vi "Abort Sequence.vi"(8 "error in (no error)":errorcluster, 10 "Sequence Name":string, 11 "Sequencing Control in":refnum<class "Sequencing Control.lvclass">) -> (0 "error out":errorcluster, 3 "Sequencing Control out":refnum<class "Sequencing Control.lvclass">)   [LabVIEW 2020, in "VolatusSeqGUI.lvlib" / "Sequencing Control.lvclass"]
uses:
  Sequencing Control.lvclass
  Sequencing Control.lvclass/Sequencing Control.ctl
  <vilib>/httpClient/LabVIEWHTTPClient.lvlib
  <vilib>/httpClient/MultipartData.ctl
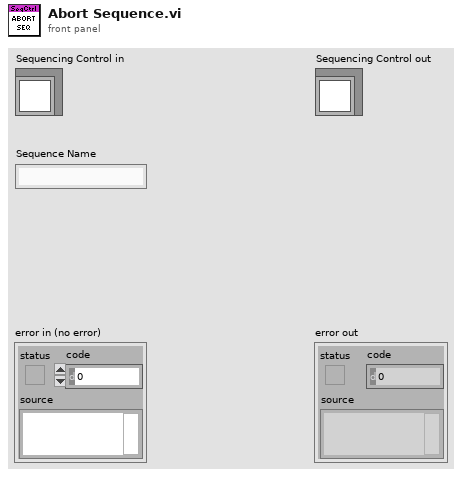
[diagram p1: front panel]
types:
  T1 = typedef "LabVIEWHTTPClient.lvlib/MultipartData.ctl" = cluster{"Name":string, "Value":string, "File":path, "Filename":string, "MIME type":string}
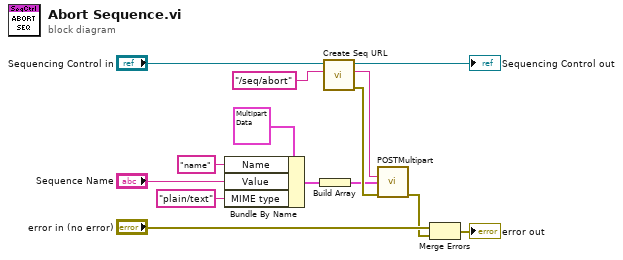
[diagram p0: block diagram]
diagram:
  n1 = Bundle By Name(cluster=T1 {"Name"="", "Value"="", "File"=path "", "Filename"="", "MIME type"="application/octet-stream"} ("Element"), "Name"="name", "Value"="Sequence Name", "MIME type"="plain/text") -> (w5:T1)
  n2 = Build Array(w5) -> (w4:T1[])
  n3 = call "Create Seq URL.vi"("Path"="/seq/abort", "Sequencing Control in"="Sequencing Control in") -> ("error out"=w14:errorcluster, "Request URL"=w2:string, "Sequencing Control out"=→"Sequencing Control out":refnum<class "Sequencing Control.lvclass">)  [unwired: 7 in]
  n4 = call <vilib>:"POSTMultipart.vi"("url"=w2, "data"=w4, "error in (no error)"=w14) -> ("error out"=w1:errorcluster)  [unwired: 9 in, 3 out]
  n5 = Merge Errors("error in (no error)", w1) -> (→"error out":errorcluster)
